vi "Motor controllers.vi"() -> ()   [LabVIEW 2016]
panel:
  in  "Control Mode":u8(ring)=2 items=["Velocity"=2, "Torque"=1]
  in  "CANOpen":T1={"termination resistor"=TRUE, "CANopen interface"=0, "baud rate"=0, "FPGA VI Reference"=refnum, "interface object out"=refnum} {"baud rate" items=["1 Mbit/s"=0, "800 kbit/s"=1, "500 kbit/s"=2, "250 kbit/s"=3, "125 kbit/s"=4, "50 kbit/s"=6, "20 kbit/s"=7, "10 kbit/s"=8]; "CANopen interface" items=["CANopen01", "CANopen02", "CANopen03", "CANopen04", "CANopen05", "CANopen06", "CANopen07", "CANopen08", "CANopen09", "CANopen10", "CANopen11", "CANopen12", "CANopen13", "CANopen14", "CANopen15", "CANopen16", "CANopen17", "CANopen18", "CANopen19", "CANopen20", "CANopen21", "CANopen22", "CANopen23", "CANopen24", "CANopen25", "CANopen26", "CANopen27", "CANopen28", "CANopen29", "CANopen30", "CANopen31", "CANopen32"]}
  in  "Node ID Right":u8=3 min=1 max=127 step=1
  in  "Node ID Left":u8=2 min=1 max=127 step=1
  # "!=="
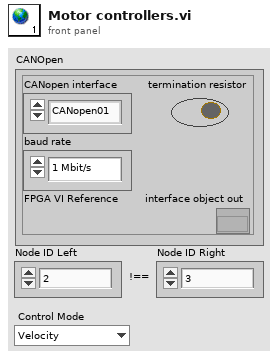
[diagram p1: front panel]
types:
  T1 = cluster{"termination resistor":bool, "CANopen interface":u32, "baud rate":u32, "FPGA VI Reference":refnum<k20>, "interface object out":refnum<k20>}
diagram:
